vi "logInCRIO.vi"(8 "error in (no error)":errorcluster, 11 "FileTransfer in":refnum<class "FileTransfer.lvclass">) -> (0 "error out":errorcluster, 3 "FileTransfer out":refnum<class "FileTransfer.lvclass">)   [LabVIEW 2016, in "FileTransfer.lvclass"]
uses:
  FileTransfer.lvclass
  FileTransfer.lvclass/FileTransfer.ctl
panel:
  out "return code 2":i32
  out "standard error 2":string
  out "standard output 2":string
  out "concatenated string":string
  out "return code":i32
  out "standard error":string
  out "standard output":string
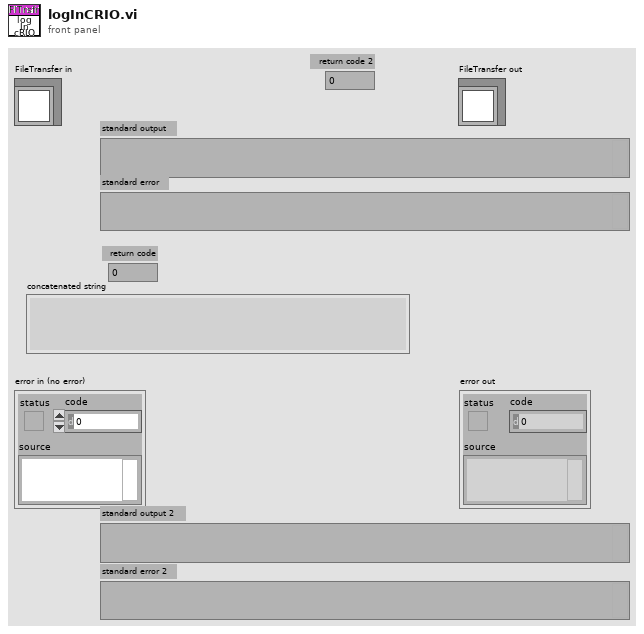
[diagram p1: front panel]
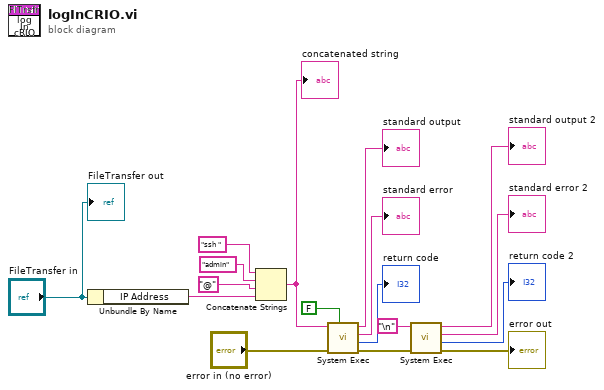
[diagram p0: block diagram]
diagram:
  n1 = Unbundle By Name("FileTransfer in") -> ("IP Address"=w14:string)
  n2 = Concatenate Strings("ssh " ("string"), "admin" ("string"), "@" ("string"), w14) -> (w13:string)
  "concatenated string" <- w13
  n3 = call <vilib>:"System Exec.vi"("wait until completion? (T)"=FALSE, "error in (no error)"="error in (no error)", "command line"=w13) -> ("error out"=w6:errorcluster, "return code"=→"return code":i32, "standard error"=→"standard error":string, "standard output"=→"standard output":string)  [unwired: 5 in]
  n4 = call <vilib>:"System Exec.vi"("error in (no error)"=w6, "command line"="\n") -> ("error out"=→"error out":errorcluster, "return code"=→"return code 2":i32, "standard error"=→"standard error 2":string, "standard output"=→"standard output 2":string)  [unwired: 6 in]
  "FileTransfer out" <- "FileTransfer in"
